vi "SendFLCam.vi"(7 "data":u16, 8 "error in (no error)":errorcluster, 9 "adadr":u8, 10 "madr":u8, 11 "board_sel":u32=1) -> (0 "error out":errorcluster)   [LabVIEW 2015, in "ESLSCDLL.lvlib"]
uses:
  ESLSCDLL.lvlib
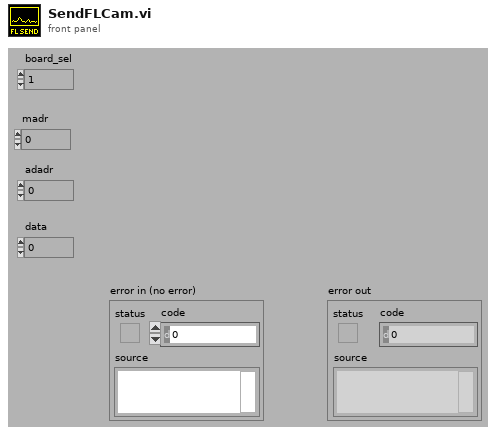
[diagram p1: front panel]
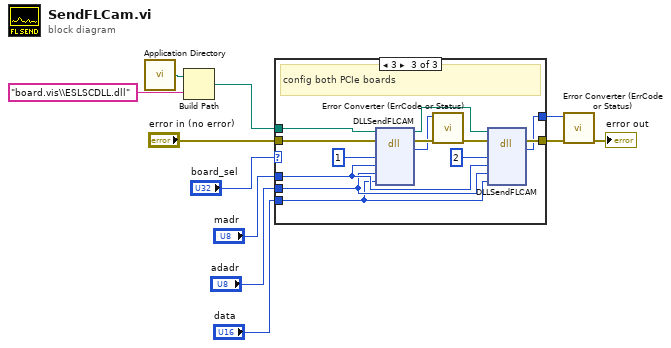
[diagram p0: block diagram]
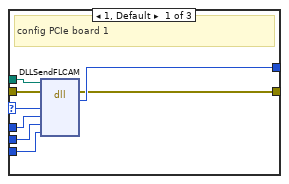
[diagram p2: hidden frame]
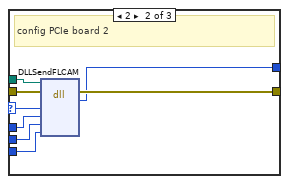
[diagram p3: hidden frame]
diagram:
  n1 = call <vilib>:"Application Directory.vi"() -> ("Application Directory"=w3:path)
  n2 = Build Path(base path=w3, name or relative path="board.vis\\ESLSCDLL.dll") -> (appended path=w1:path)
  n3 = case shown="3" "board_sel" {
    selector: "board_sel" -> [w19 w27 _]
    tunnel: "madr" -> [w18 w26 w38]
    tunnel: "adadr" -> [w17 w25 w37]
    tunnel: "data" -> [w16 w24 w36]
    tunnel: "error in (no error)" -> [w12 w20 w35]
    tunnel: [w14 w23 w31] -> w5
    tunnel: [w15 w22 w30] -> w4
    tunnel: w1 -> [w13 w21 w29]
    frame 1, Default {
      # "config PCIe board 1"
      n4 = dll-call lib="C:/ENTW/PCIE/LV64/board.vis/ESLSCDLL.dll" fn="DLLSendFLCAM" ("lwlscdll.dll:DLLSetADAmpRed")(path in=w13, error in=w12, "drv"=w19, "madr"=w18, "adadr"=w17, "data"=w16) -> (error out=w14:errorcluster, "es_status_codes"=w15:i32)  [unwired: 5 in, 1 out]
    }
    frame 2 {
      # "config PCIe board 2"
      n5 = dll-call lib="C:/ENTW/PCIE/LV64/board.vis/ESLSCDLL.dll" fn="DLLSendFLCAM" ("lwlscdll.dll:DLLSetADAmpRed")(path in=w21, error in=w20, "drv"=w27, "madr"=w26, "adadr"=w25, "data"=w24) -> (error out=w23:errorcluster, "es_status_codes"=w22:i32)  [unwired: 5 in, 1 out]
    }
    frame 3 {
      # "config both PCIe boards"
      n6 = dll-call lib="C:/ENTW/PCIE/LV64/board.vis/ESLSCDLL.dll" fn="DLLSendFLCAM" ("lwlscdll.dll:DLLSetADAmpRed")(path in=w29, error in=w35, "drv"=u32 1, "madr"=w38, "adadr"=w37, "data"=w36) -> (path out=w28:path, error out=w34:errorcluster, "es_status_codes"=w33:i32)  [unwired: 5 in]
      n7 = call "Error Converter (ErrCode or Status).vi"("error in (no error)"=w34, "error code"=w33) -> ("error out"=w32:errorcluster)  [unwired: 9 in]
      n8 = dll-call lib="C:/ENTW/PCIE/LV64/board.vis/ESLSCDLL.dll" fn="DLLSendFLCAM" ("lwlscdll.dll:DLLSetADAmpRed")(path in=w28, error in=w32, "drv"=u32 2, "madr"=w38, "adadr"=w37, "data"=w36) -> (error out=w31:errorcluster, "es_status_codes"=w30:i32)  [unwired: 5 in, 1 out]
    }
  }
  n9 = call "Error Converter (ErrCode or Status).vi"("error in (no error)"=w5, "error code"=w4) -> ("error out"=→"error out":errorcluster)  [unwired: 9 in]
